vi "PPR_DRIVE_EXECUTE.vi"(6 "Pass_Through_Time":dbl=-1.0 format="%33.4f", 8 "error in (no error)":errorcluster) -> (0 "error out":errorcluster)   [LabVIEW 2019]
uses:
  <vilib>/Rock Robotics/WPI/ThirdParty/JAS_Junk/TrajLib/VI/BoolCmd_Recv_Internal.vi
  <vilib>/Rock Robotics/WPI/ThirdParty/JAS_Junk/TrajLib/VI/numCmd_ObtainQueue_TwoDbl.vi
  <vilib>/Rock Robotics/WPI/ThirdParty/JAS_Junk/TrajLib/VI/Util_GetTime_U32.vi
  <vilib>/Rock Robotics/WPI/ThirdParty/JAS_Junk/TrajLib/MathUtil_InputModulus.vi
  <vilib>/Rock Robotics/WPI/ThirdParty/JAS_Junk/TrajLib/VI/BoolCmd_ObtainQueue.vi
  <vilib>/Rock Robotics/WPI/ThirdParty/JAS_Junk/TrajLib/VI/Util_GetTime_U64.vi
  PPR_DRIVE_GLOBALS.vi
  <vilib>/Rock Robotics/WPI/ThirdParty/JAS_Junk/TrajLib/Trajectory_Library.lvlib
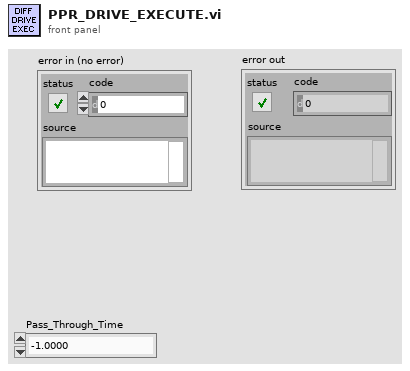
[diagram p1: front panel]
types:
  T1 = typedef "PPR_DRIVE_Wheel_TYPDEF.ctl" = cluster{"Drive Motor":T2, "Wheel Encoder":T7}
  T2 = typedef "WPI_MotorControlDeviceRef.ctl" = cluster{"DeviceStatus":errorcluster, "Type":T3, "PWM":cluster{"PWM Channel":T4, "DeadBand":T5}, "CAN":cluster{"Device Number":u8, "SetOutput VI Ref":variant, "GetOutput VI Ref":variant, "Enable VI Ref":variant, "Disable VI Ref":variant, "Data":variant}, "Invert":bool, "DIO PWM":cluster{"PWM \"Enable\" Channel":T4, "DIOChannel":T6, "PWM Rate":dbl}}
  T3 = typedef "WPI_MotorControlType.ctl" = enum16{"PWM", "CAN", "DIO PWM"}
  T4 = typedef "FPGA_DIOPWMChannel.ctl" = enum8{"PWM 0", "PWM 1", "PWM 2", "PWM 3", "PWM 4", "PWM 5", "PWM 6", "PWM 7", "PWM 8", "PWM 9", "PWM MXP 0", "PWM MXP 1", "PWM MXP 2", "PWM MXP 3", "PWM MXP 4", "PWM MXP 5", "PWM MXP 6", "PWM MXP 7", "PWM MXP 8", "PWM MXP 9", "Invalid"}
  T5 = typedef "WPI_PWMDeadband.ctl" = cluster{"Name":string, "maxPositivePwm":i32, "minPositivePwm":i32, "centerPwm":i32, "maxNegativePwm":i32, "minNegativePwm":i32, "angularRange":u16}
  T6 = typedef "FPGA_DIOChannel.ctl" = enum8{"DIO 0", "DIO 1", "DIO 2", "DIO 3", "DIO 4", "DIO 5", "DIO 6", "DIO 7", "DIO 8", "DIO 9", "DIO MXP 0", "DIO MXP 1", "DIO MXP 2", "DIO MXP 3", "DIO MXP 4", "DIO MXP 5", "DIO MXP 6", "DIO MXP 7", "DIO MXP 8", "DIO MXP 9", "DIO MXP 10", "DIO MXP 11", "DIO MXP 12", "DIO MXP 13", "DIO MXP 14", "DIO MXP 15", "SPI Port CS1", "SPI Port CS2", "SPI Port CS3", "SPI Port MISO", "SPI Port MOSI", "Invalid"}
  T7 = typedef "WPI_EncoderDevRef.ctl" = cluster{"DevStatus":errorcluster, "EncoderIndex":T8, "CounterIndex":T9, "DistancePerCount":dbl, "Decoding Type":T10}
  T8 = typedef "FPGA_EncoderIdx.ctl" = enum8{"Enc 0", "Enc 1", "Enc 2", "Enc 3", "Enc 4", "Enc 5", "Enc 6", "Enc 7", "Invalid"}
  T9 = typedef "FPGA_CounterCtrSystemIndex.ctl" = enum8{"Ctr 0", "Ctr 1", "Ctr 2", "Ctr 3", "Ctr 4", "Ctr 5", "Ctr 6", "Ctr 7", "Invalid"}
  T10 = typedef "WPI_EncoderType.ctl" = enum16{"1x", "2x", "4x"}
  T11 = typedef "WPI_GyroDevRef.ctl" = cluster{"DevStatus":errorcluster, "Analog Channel":T12, "Gain (VoltsPerDegree/Second)":dbl, "Gyro Type":enum16{"Analog", "XRS450"}, "Handle":i32, "SPI Bus":T13, "Device Found":bool, "Sample Rate":dbl, "Calibrate On Open":bool, "Offset":dbl}
  T12 = typedef "FPGA_AIChannel.ctl" = enum8{"AI 0", "AI 1", "AI 2", "AI 3", "AI MXP 0", "AI MXP 1", "AI MXP 2", "AI MXP 3", "Invalid"}
  T13 = typedef "spi_bus.ctl" = enum16{"SPI On-Board, CS0", "SPI On-Board, CS1", "SPI On-Board, CS2", "SPI On-Board, CS3", "SPI MXP", "Invalid"}
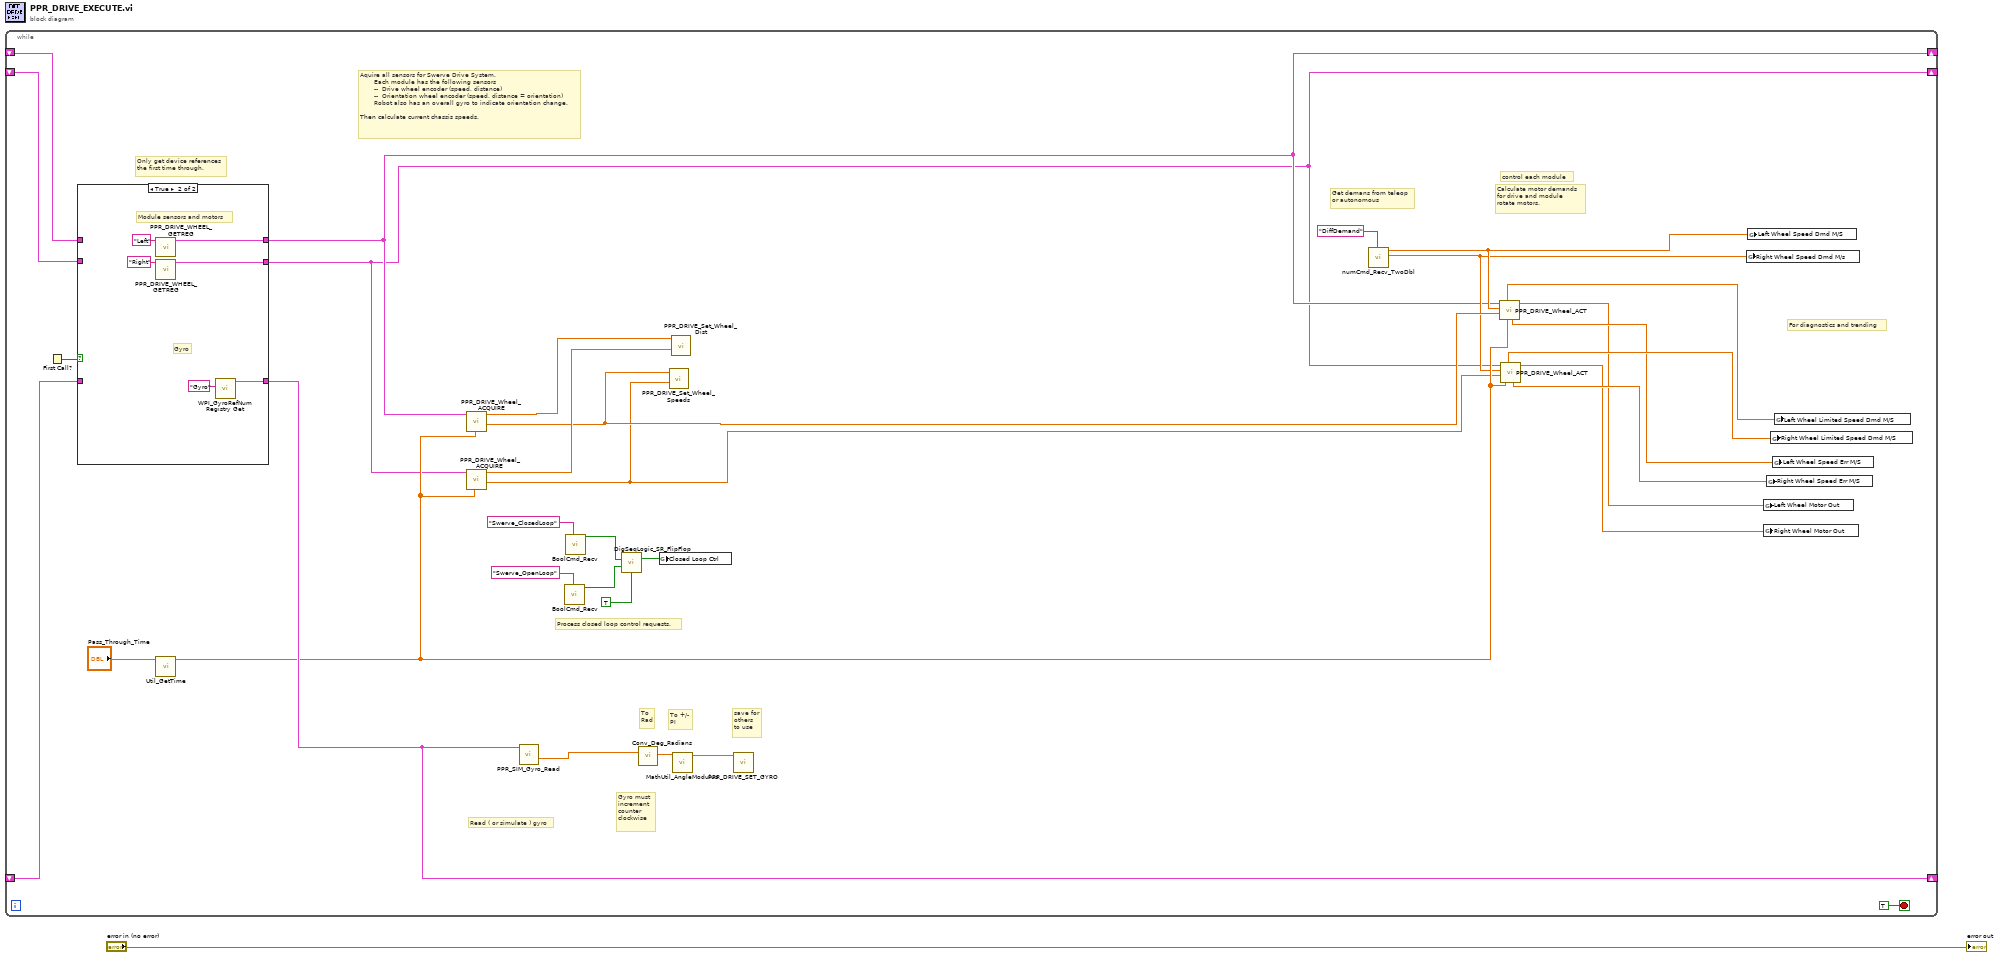
[diagram p0: block diagram]
diagram:
  n1 = while {
    shift-right: [w5] -> _
    shift-left: _ -> [w4]
    shift-right: [w26] -> _
    shift-left: _ -> [w25]
    shift-right: [w3] -> _
    shift-left: _ -> [w2]
    stop <- TRUE stop-if-true
    # "Process closed loop control requests."
    # "Only get device references\nthe first time through."
    # "save for\nothers\nto use"
    # "For diagnostics and trending"
    # "Gyro must\nincrement \ncounter\nclockwise"
    # "To +/-\nPI"
    # "To\nRad"
    # "Read ( or simulate ) gyro"
    # "Aquire all sensors for Swerve Drive System.\n       Each module has the following sensors\n       --  Drive wheel encoder (speed, distance)\n       --  Orientation wheel encoder (speed, distance = orientation)\n       Robot also has an overall gyro to indicate orientation change.\n\nThen calculate current chassis speeds."
    # "Calculate motor demands\nfor drive and module \nrotate motors."
    # "Get demans from teleop\nor autonomous"
    # "control each module"
    n2 = First Call?() -> (First Call?: T/F=w27:bool)
    n3 = case shown="True" w27 {
      tunnel: [w36 w42] -> w26
      tunnel: w25 -> [w36 _]
      tunnel: [w35 w38] -> w5
      tunnel: [w34 w37] -> w3
      tunnel: w4 -> [w35 _]
      tunnel: w2 -> [w34 _]
      frame False {
      }
      frame True {
        # "Module sensors and motors"
        # "Gyro"
        n4 = call "PPR_DRIVE_WHEEL_GETREG.vi"("Side"="Left") -> ("Diff Wheel TypDef"=w38:T1)  [unwired: 10 in]
        n5 = call "PPR_DRIVE_WHEEL_GETREG.vi"("Side"="Right") -> ("Diff Wheel TypDef"=w37:T1)  [unwired: 10 in]
        n6 = call <vilib>:"WPI_GyroRefNum Registry Get.vi"("refnum name"="Gyro") -> ("GyroDevRef"=w42:T11)  [unwired: 9 in, 1 out]
      }
    }
    n7 = call <vilib>:"Util_GetTime.vi"("Pass_Through_Time"="Pass_Through_Time") -> ("FPGA_Time_Seconds"=w24:dbl)  [unwired: 8 in, 2 out]
    n8 = call "PPR_DRIVE_Wheel_ACQUIRE.vi"("Pass_Through_Time"=w24, "Diff Drive Wheel TypDef"=w3) -> ("Speed M/S"=w14:dbl, "Distance M"=w16:dbl)  [unwired: 8 in]
    n9 = call "PPR_DRIVE_Wheel_ACQUIRE.vi"("Pass_Through_Time"=w24, "Diff Drive Wheel TypDef"=w5) -> ("Speed M/S"=w15:dbl, "Distance M"=w17:dbl)  [unwired: 8 in]
    n10 = call "PPR_SIM_Gyro_Read.vi"("GyroDevRef"=w26) -> ("Gyro_Cont_Deg"=w30:dbl)  [unwired: 10 in]
    n11 = call <vilib>:"BoolCmd_Recv.vi"("Command Name"="Swerve_OpenLoop") -> ("New Request"=w20:bool)  [unwired: 9 in, 1 out]
    n12 = call <vilib>:"BoolCmd_Recv.vi"("Command Name"="Swerve_ClosedLoop") -> ("New Request"=w21:bool)  [unwired: 9 in, 1 out]
    n13 = call <vilib>:"DigSeqLogic_SR_FlipFlop.vi"("Set"=w21, "Reset"=w20, "Initial Value"=TRUE) -> ("Output"=w18:bool)  [unwired: 11 in, 1 out]
    n14 = call <vilib>:"Conv_Deg_Radians.vi"("Degress"=w30) -> ("Radians"=w31:dbl)  [unwired: 10 in]
    n15 = global write "PPR_DRIVE_GLOBALS.vi" "Closed Loop Ctrl"(w18) -> ()
    n16 = call "PPR_DRIVE_Set_Wheel_Speeds.vi"("Right Wheel Speed M/S"=w14, "Left Wheel Speed M/S"=w15) -> ()  [unwired: 10 in]
    n17 = call "PPR_DRIVE_Set_Wheel_Dist.vi"("Right Wheel Dist M"=w16, "Left Wheel Dist M"=w17) -> ()  [unwired: 10 in]
    n18 = call <vilib>:"MathUtil_AngleModulus.vi"("InputAngle"=w31) -> ("ModulsAngle"=w29:dbl)  [unwired: 10 in]
    n19 = call "PPR_DRIVE_SET_GYRO.vi"("Gyro Heading Radians"=w29) -> ()  [unwired: 11 in]
    n20 = call <vilib>:"numCmd_Recv_TwoDbl.vi"("Command Name"="DiffDemand") -> ("Value 2"=w6:dbl, "Value 1"=w7:dbl)  [unwired: 7 in, 2 out]
    n21 = call "PPR_DRIVE_Wheel_ACT.vi"("Pass_Through_Time"=w24, "Wheel Speed M/S"=w15, "Wheel Speed Dmd M/S"=w7, "Diff Wheel TypDef"=w5) -> ("Wheel Motor Dmd"=w9:dbl, "WheelSpeedErr"=w11:dbl, "Limited Speed Dmd M/S"=w13:dbl)  [unwired: 5 in]
    n22 = call "PPR_DRIVE_Wheel_ACT.vi"("Pass_Through_Time"=w24, "Wheel Speed M/S"=w14, "Wheel Speed Dmd M/S"=w6, "Diff Wheel TypDef"=w3) -> ("Wheel Motor Dmd"=w8:dbl, "WheelSpeedErr"=w10:dbl, "Limited Speed Dmd M/S"=w12:dbl)  [unwired: 5 in]
    n23 = global write "PPR_DRIVE_GLOBALS.vi" "Right Wheel Speed Dmd M/s"(w6) -> ()
    n24 = global write "PPR_DRIVE_GLOBALS.vi" "Left Wheel Speed Dmd M/S"(w7) -> ()
    n25 = global write "PPR_DRIVE_GLOBALS.vi" "Right Wheel Motor Out"(w8) -> ()
    n26 = global write "PPR_DRIVE_GLOBALS.vi" "Left Wheel Motor Out"(w9) -> ()
    n27 = global write "PPR_DRIVE_GLOBALS.vi" "Right Wheel Speed Err M/S"(w10) -> ()
    n28 = global write "PPR_DRIVE_GLOBALS.vi" "Right Wheel Limited Speed Dmd M/S"(w12) -> ()
    n29 = global write "PPR_DRIVE_GLOBALS.vi" "Left Wheel Speed Err M/S"(w11) -> ()
    n30 = global write "PPR_DRIVE_GLOBALS.vi" "Left Wheel Limited Speed Dmd M/S"(w13) -> ()
  }
  "error out" <- "error in (no error)"
